vi "Prog_Status_Handler.vi"(1 "Status Cluster":T2, 3 "Simulate/Run":T1) -> ()   [LabVIEW 2015]
uses:
  Gen Trav/Status_Cluster.ctl
  Gen Trav/Multi_Run_Status.ctl
  Controls/User_Specific_mode.ctl
  Globals/Trav_pos_global.vi
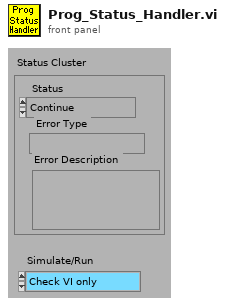
[diagram p1: front panel]
types:
  T1 = typedef "User_Specific_mode.ctl" = enum16{"Check VI only", "Run VI"}
  T2 = typedef "Status_Cluster.ctl" = cluster{"Status":T3, "Error Type":string, "Error Description":string}
  T3 = typedef "Multi_Run_Status.ctl" = enum16{"Continue", "Jump to Next Point", "Jump to Next Row", "Jump To Fall Back", "Terminate Run"}
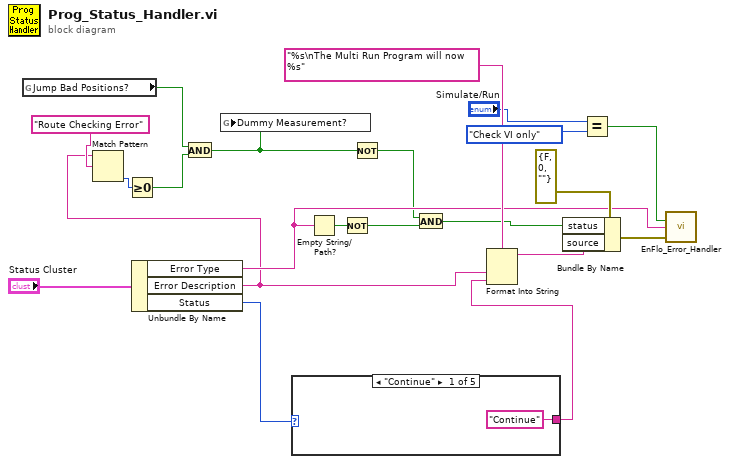
[diagram p0: block diagram]
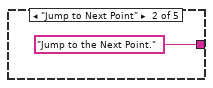
[diagram p2: hidden frame]
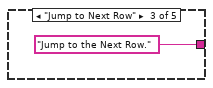
[diagram p3: hidden frame]
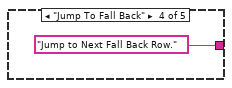
[diagram p4: hidden frame]
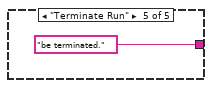
[diagram p5: hidden frame]
diagram:
  n1 = global read "Trav_pos_global.vi" "Jump Bad Positions?"() -> (w5:bool)
  n2 = Unbundle By Name("Status Cluster") -> ("Error Type"=w10:string, "Error Description"=w7:string, "Status"=w14:T3)
  n3 = Match Pattern(string=w7, regular expression="Route Checking Error") -> (offset past match=w8:i32)  [unwired: 4 out]
  n4 = Greater Or Equal To 0?(x=w8) -> (x >= 0?=w6:bool)
  n5 = And(x=w5, y=w6) -> (x .and. y?=w1:bool)
  n6 = global write "Trav_pos_global.vi" "Dummy Measurement?"(w1) -> ()
  n7 = case shown="\"Continue\"" w14 {
    tunnel: ["Continue" "Jump to the Next Point." "Jump to the Next Row." "Jump to Next Fall Back Row." "be terminated."] -> w21
    frame "Continue" {
    }
    frame "Jump to Next Point" {
    }
    frame "Jump to Next Row" {
    }
    frame "Jump To Fall Back" {
    }
    frame "Terminate Run" {
    }
  }
  n8 = Empty String/Path?(string/path=w10) -> (empty?=w13:bool)
  n9 = Not(x=w13) -> (.not. x?=w4:bool)
  n10 = Not(x=w1) -> (.not. x?=w2:bool)
  n11 = And(x=w2, y=w4) -> (x .and. y?=w3:bool)
  n12 = Format Into String(format string="%s\nThe Multi Run Program will now %s" ("Format String"), w7, w21) -> (resulting string=w16:string)  [unwired: 2 in, 1 out]
  n13 = Bundle By Name(cluster=errorcluster {"status"=FALSE, "code"=0, "source"=""} ("error in (no error)"), "status"=w3, "source"=w16) -> (w19:errorcluster)
  n14 = Equal?(x="Simulate/Run", y=User_Specific_mode."Check VI only" ("Simulate/Run")) -> (x = y?=w17:bool)
  n15 = call "EnFlo_Error_Handler.vi"("error in (no error)"=w19, "Error Type"=w10, "Dialog Box (T)"=w17) -> ()  [unwired: 3 out]
